vi "Simple Temperature Controller.vi"() -> ()   [LabVIEW 2013]
uses:
  Heating.ctl
  <vilib>/Analysis/baseanly.llb/Mean (DBL).vi
  <vilib>/Analysis/NI_AALBase.lvlib
panel:
  out "Heating?":T1
  in  "Temperature Control":dbl(slide) scale=0.0..2500.0
  out "Mean":dbl format="%0.2f"
  out "Current Mean":dbl
  out "Current Temperature":dbl
  out "Min value":dbl
  out "Max value":dbl
  in  "Stop Button":bool
  out "History":dbl(graph)
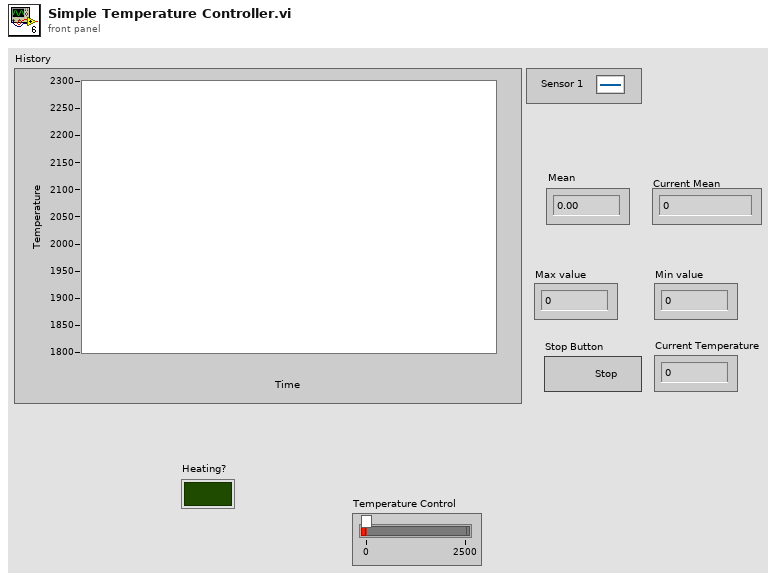
[diagram p1: front panel]
types:
  T1 = typedef "Heating.ctl" = bool
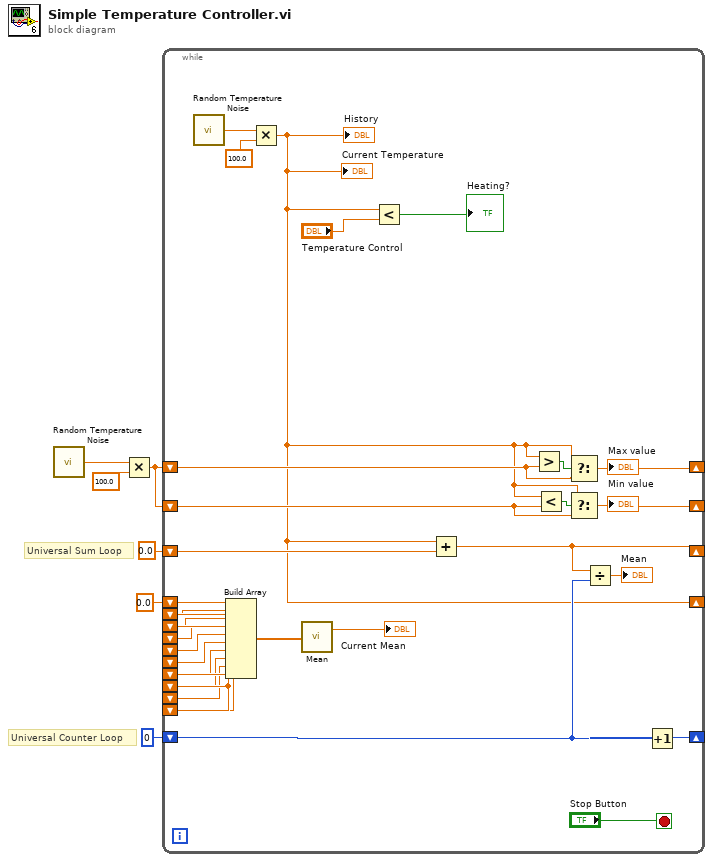
[diagram p0: block diagram]
diagram:
  w1 = 0.0
  # "Universal Sum Loop"
  # "Universal Counter Loop"
  n1 = call "Random Temperature Noise.vi"() -> ("Temperature"=w5:dbl)  [unwired: 1 in]
  n2 = Multiply(x=w5, y=100.0) -> (x*y=w3:dbl)
  n3 = while {
    shift-right: [w10] -> _
    shift-left: 0.0 -> [w14]
    shift-right: [w30] -> _
    shift-left: w3 -> [w28]
    shift-right: [w29] -> _
    shift-left: w3 -> [w27]
    shift-right: [w9] -> _
    shift-left: w1 -> [w24]
    shift-left: w1 -> [w23]
    shift-left: w1 -> [w15]
    shift-left: w1 -> [w22]
    shift-left: w1 -> [w17]
    shift-left: w1 -> [w18]
    shift-right: [w25] -> _
    shift-left: 0 -> [w11]
    shift-left: w1 -> [w16]
    shift-left: w1 -> [w21]
    shift-left: w1 -> [w19]
    shift-left: w1 -> [w20]
    stop <- "Stop Button" stop-if-true
    n4 = call "Random Temperature Noise.vi"() -> ("Temperature"=w33:dbl)  [unwired: 1 in]
    n5 = Build Array(w24, w23, w22, w21, w20, w19, w18, w17, w16, w15) -> (w8:dbl[])
    n6 = Multiply(x=w33, y=100.0) -> (x*y=w9:dbl)
    "History" <- w9
    "Current Temperature" <- w9
    n7 = call-poly <vilib>:"Mean.vi"("X"=w8) -> ("mean"=→"Current Mean":dbl)  [unwired: 1 out]
    n8 = Less?(x=w9, y="Temperature Control") -> (x < y?=→"Heating?":bool)
    n9 = Add(x=w9, y=w14) -> (x+y=w10:dbl)
    n10 = Greater?(x=w9, y=w28) -> (0:w32:bool)
    n11 = Less?(x=w9, y=w27) -> (x < y?=w31:bool)
    n12 = Select(t=w9, s=w32, f=w28) -> (s? t:f=w30:dbl)
    "Max value" <- w30
    n13 = Select(t=w9, s=w31, f=w27) -> (s? t:f=w29:dbl)
    "Min value" <- w29
    n14 = Divide(x=w10, y=w11) -> (x/y=→"Mean":dbl)
    n15 = Increment(x=w11) -> (x+1=w25:i32)
  }
